vi "GetEnvironmentParams - Test.vi"() -> ()   [LabVIEW 2017]
uses:
  AT901 API/Structures/Struct EnvironmentData.ctl
panel:
  out "Environmental Data":T1
  out "error out":errorcluster
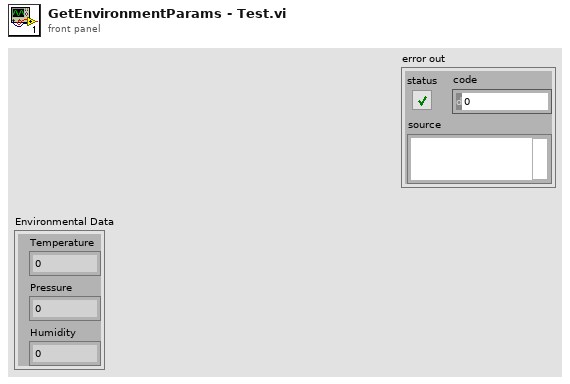
[diagram p1: front panel]
types:
  T1 = typedef "Struct EnvironmentData.ctl" = cluster{"Temperature":dbl, "Pressure":dbl, "Humidity":dbl}
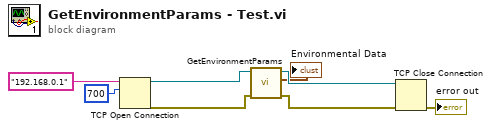
[diagram p0: block diagram]
diagram:
  n1 = TCP Open Connection(address="192.168.0.1", remote port or service name=u16 700) -> (connection ID=w5:refnum<k5>, error out=w2:errorcluster)  [unwired: 3 in]
  n2 = call "GetEnvironmentParams.vi"("error in (no error)"=w2, "TCP Network Connection in"=w5) -> ("error out"=w3:errorcluster, "Environmental Data"=→"Environmental Data":T1, "TCP Network Connection out"=w4:refnum<k5>)  [unwired: 5 in, 2 out]
  n3 = TCP Close Connection(connection ID=w4, error in (no error)=w3) -> (error out=→"error out":errorcluster)  [unwired: 1 in, 1 out]
